vi "MuStLiMo_si_initialize.vi"(1 "Target Pulse Duration (ms)":dbl=2000.0, 2 "Target Position (decimicrons)":dbl=180000.0) -> ()   [LabVIEW 2014]
doc: "This example shows a single axis straight-line move using the NI SoftMotion Line function block.\n\nNote: You must have the LabVIEW NI SoftMotion Module installed to run this example."
uses:
  <vilib>/Motion/Express/_s/nimc.fb.read.readExecutionData.axis.vi
  <vilib>/Motion/Express/_s/nimc.fb.straightLineMove.startStraightLineMove.axis.modeAbsolute.0.vi
  <vilib>/Motion/Express/_s/nimc.fb.stopMove.stop.axis.modeDecelerate.vi
  <vilib>/Motion/BlockNode/FB.NIMotion.xnode
panel:
  out "Numeric":i32
  out "Acceleration (decimicrons/s2)":dbl
  out "Velocity (decimicrons/s)":dbl
  out "Distance (decimicrons)":dbl
  out "error out":errorcluster={"status"=FALSE, "code"=77003, "source"="Invoke Node in nimc.fb.straightLineMove.startStraightLineMove.axis.modeAbsolute.0.vi:5060005->Multiple Straight Line Moves.vi"}
  in  "Resource":refnum<k21>="Axis 1"
  # "Target Parameters"
  # "Computed Inputs"
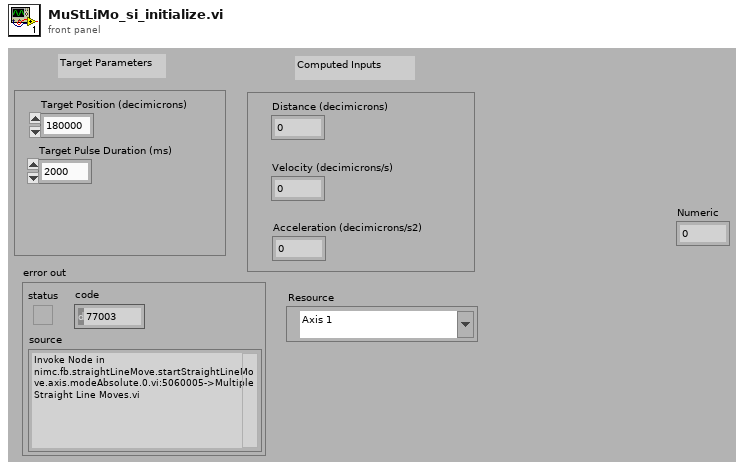
[diagram p1: front panel]
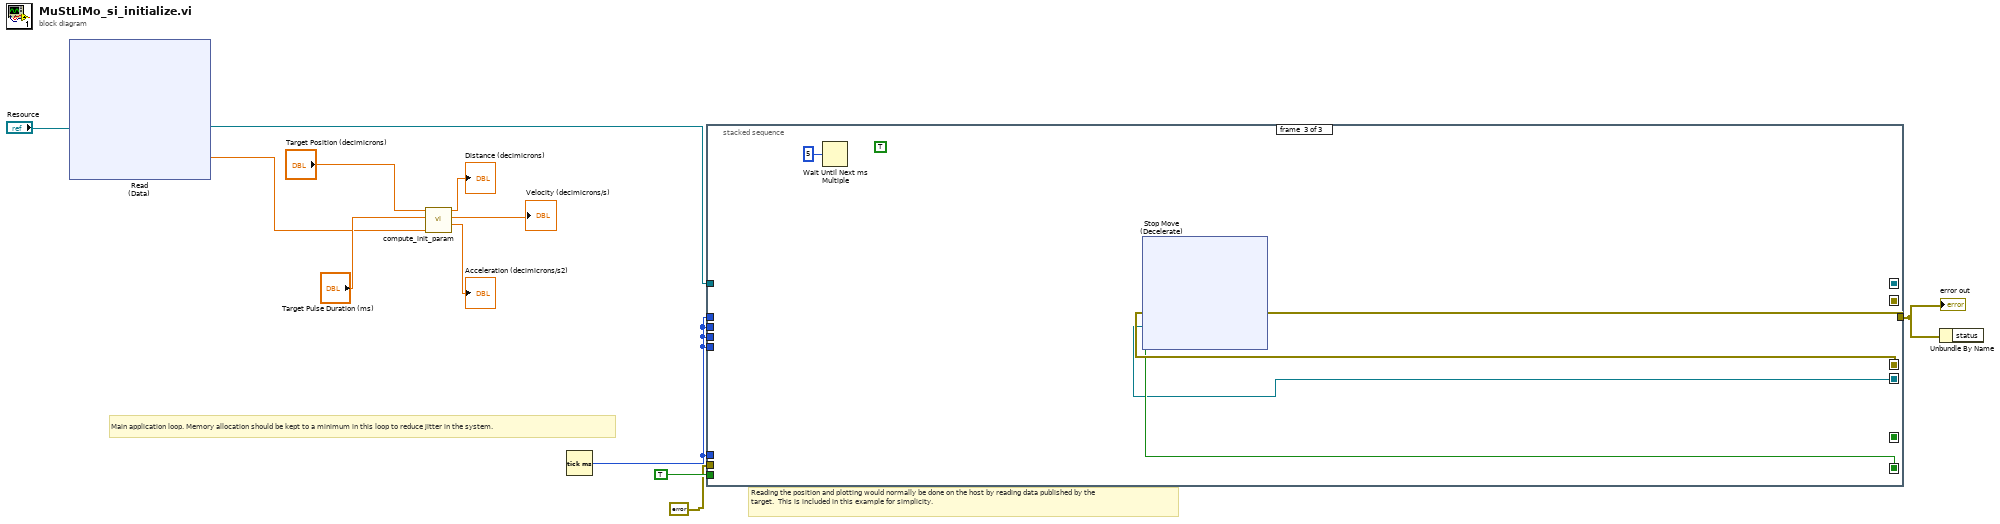
[diagram p0: block diagram]
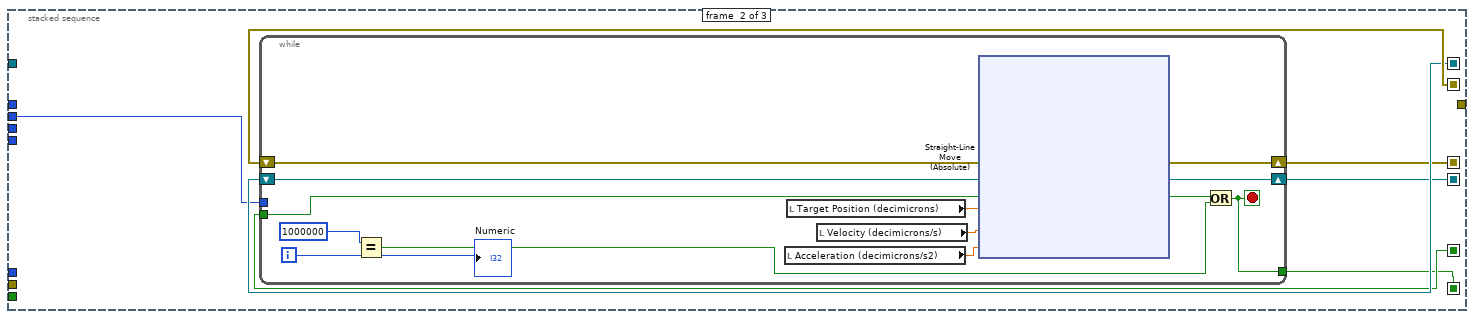
[diagram p3: hidden frame]
diagram:
  # "Reading the position and plotting would normally be done on the host by reading data published by the target.  This is included in this example for simplicity."
  # "Main application loop. Memory allocation should be kept to a minimum in this loop to reduce jitter in the system."
  n1 = xnode "Read\n(Data)"("resource"="Resource") -> ("resource out"=w4:refnum<k21>, "position"=w6:dbl)  [unwired: 1 in, 3 out]
  n2 = call "compute_init_param.vi"("Current Position (decimicrons)"=w6, "Target Pulse Duration (ms)"="Target Pulse Duration (ms)", "Target Position (decimicrons)"="Target Position (decimicrons)") -> ("Acceleration (decimicrons/s2)"=→"Acceleration (decimicrons/s2)":dbl, "Velocity (decimicrons/s)"=→"Velocity (decimicrons/s)":dbl, "Distance (decimicrons)"=→"Distance (decimicrons)":dbl)  [unwired: 6 in]
  n3 = Tick Count (ms)() -> (millisecond timer value=w11:u32)
  n4 = stacked-sequence {
    seq-local: [w13 _ _] -> [_ w22 _]
    seq-local: [w14 _ _] -> [_ w21 _]
    seq-local: [w15 _ _] -> [_ w18 _]
    seq-local: [_ w20 _] -> [_ _ w56]
    seq-local: [_ w19 _] -> [_ _ w54]
    seq-local: [_ w16 _] -> [_ _ w55]
    tunnel: w4 -> [w14 _ _]
    tunnel: errorcluster {"status"=FALSE, "code"=0, "source"=""} ("Error") -> [w13 _ _]
    tunnel: TRUE ("approach forward") -> [w15 _ _]
    tunnel: w11 -> [_ _ _]
    tunnel: w11 -> [_ w17 _]
    tunnel: w11 -> [_ _ _]
    tunnel: w11 -> [_ _ _]
    tunnel: [_ _ w53] -> w2
    tunnel: w11 -> [_ _ _]
    frame #0 {
    }
    frame #1 {
      n5 = while {
        tunnel: w18 -> [w32]
        tunnel: w17 -> [_]
        shift-right: [w34] -> w20
        shift-left: w22 -> [w28]
        shift-right: [w33] -> w19
        shift-left: w21 -> [w35]
        tunnel: [w23] -> w16
        i -> [w25]
        stop <- w23 stop-if-true
        n6 = Equal?(x=1000000, y=w25) -> (x = y?=w24:bool)
        n7 = local read "Acceleration (decimicrons/s2)"() -> (w29:dbl)
        n8 = local read "Target Position (decimicrons)"() -> (w31:dbl)
        n9 = local read "Velocity (decimicrons/s)"() -> (w30:dbl)
        n10 = xnode "Straight-Line Move\n(Absolute)"("error in"=w28, "resource"=w35, "execute"=w32, "position"=w31, "velocity"=w30, "acceleration"=w29) -> ("error out"=w34:errorcluster, "resource out"=w33:refnum<k21>, "done"=w27:bool)
        n11 = Or(x=w27, y=w24) -> (x .or. y?=w23:bool)
        "Numeric" <- w25
      }
    }
    frame #2 {
      (unwired) TRUE
      n12 = Wait Until Next ms Multiple(millisecond multiple=u32 5) -> ()  [unwired: 1 out]
      n13 = xnode "Stop Move\n(Decelerate)"("error in"=w56, "resource"=w54, "execute"=w55) -> ("error out"=w53:errorcluster)  [unwired: 1 out]
    }
  }
  "error out" <- w2
  n14 = Unbundle By Name(w2) -> ()  [unwired: 1 out]
